vi "Refresh Config Data from UDP.vi"(8 "error in (no error)":errorcluster, 10 "Timeout (2s)":dbl=2.0, 11 "Ethernet in":refnum<class "ENET_BS120x.lvclass">) -> (0 "error out":errorcluster, 1 "Received":bool, 2 "Configuration Data":string, 3 "Ethernet out":refnum<class "ENET_BS120x.lvclass">)   [LabVIEW 2021, in "BS120x Driver.lvlib" / "ENET_BS120x.lvclass"]
uses:
  ENET_BS120x.lvclass
  ENET_BS120x.lvclass/ENET_BS120x.ctl
panel:
  out "Array":string[](array[string])
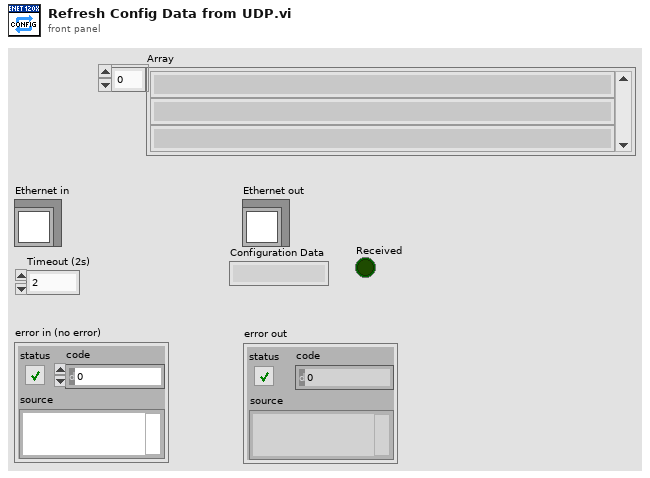
[diagram p1: front panel]
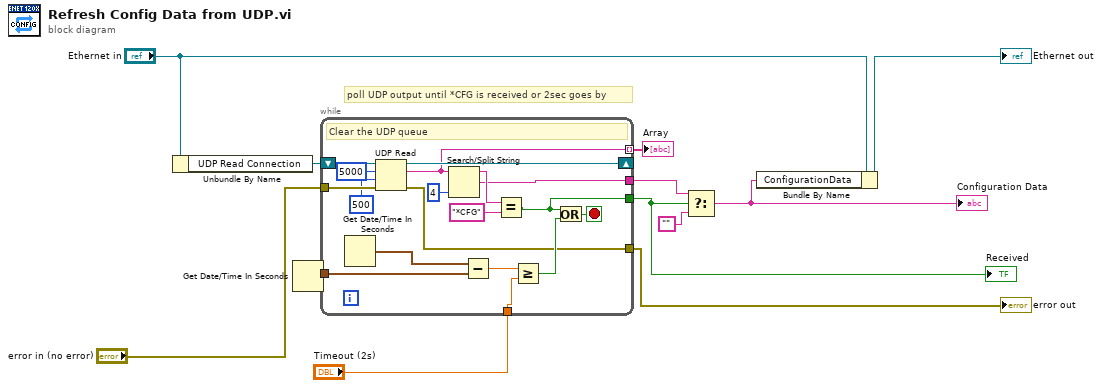
[diagram p0: block diagram]
diagram:
  # "poll UDP output until *CFG is received or 2sec goes by"
  n1 = Unbundle By Name("Ethernet in") -> ("UDP Read Connection"=w12:refnum<k16>)
  n2 = Get Date/Time In Seconds() -> (seconds since 1Jan1904=w8:timestamp)
  n3 = while {
    shift-right: [w28] -> _
    shift-left: w12 -> [w29]
    tunnel: "error in (no error)" -> [w30]
    tunnel: [w15] -> w6
    tunnel: w8 -> [w24]
    tunnel: [w16] -> w7
    tunnel: [w20] -> w3
    tunnel: "Timeout (2s)" -> [w19]
    tunnel: [w14] -> w1 mode=indexing
    stop <- w22 stop-if-true
    # "Clear the UDP queue"
    n4 = Get Date/Time In Seconds() -> (seconds since 1Jan1904=w25:timestamp)
    n5 = UDP Read(connection ID=w29, max size (548)=5000, timeout ms (25000)=500, 8:w30) -> (data out=w14:string, error out=w20:errorcluster, 3:w28:refnum<k16>)  [unwired: 2 out]
    n6 = Search/Split String(string=w14, offset (0)=4) -> (substring before match=w18:string, match + rest of string=w15:string)  [unwired: 1 in, 1 out]
    n7 = Subtract(x=w25, y=w24) -> (x-y=w23:dbl)
    n8 = Equal?(x=w18, y="*CFG") -> (x = y?=w16:bool)
    n9 = Greater Or Equal?(x=w23, y=w19) -> (x >= y?=w21:bool)
    n10 = Or(x=w16, y=w21) -> (x .or. y?=w22:bool)
  }
  "error out" <- w3
  "Received" <- w7
  "Array" <- w1
  n11 = Select(t=w6, s=w7, f="") -> (s? t:f=w4:string)
  "Configuration Data" <- w4
  n12 = Bundle By Name(cluster="Ethernet in", "ConfigurationData"=w4) -> (→"Ethernet out":refnum<class "ENET_BS120x.lvclass">)
